vi "database_path.vi"(10 "部位":string, 11 "产品序号":string) -> (2 "database path":path)   [LabVIEW 2018]
panel:
  out "添加的路径":path
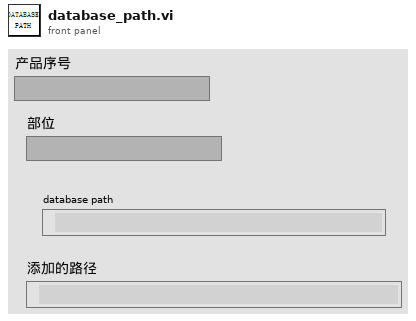
[diagram p1: front panel]
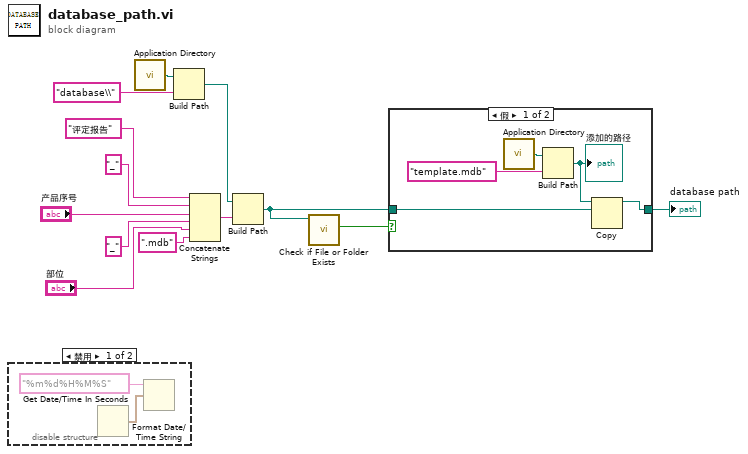
[diagram p0: block diagram]
diagram:
  n1 = disable-structure shown="禁用" {
    frame Disabled {
      n2 = Get Date/Time In Seconds() -> (seconds since 1Jan1904=w15:timestamp)
      n3 = Format Date/Time String(time format string (%c)="%m%d%H%M%S" ("时间格式字符串(%c)"), seconds (now)=w15) -> ()  [unwired: 1 in, 1 out]
    }
    frame Enabled {
    }
  }
  n4 = call <vilib>:"Application Directory.vi"() -> ("Application Directory"=w10:path)
  n5 = Build Path(base path=w10, name or relative path="database\\" ("名称或相对路径")) -> (appended path=w8:path)
  n6 = Concatenate Strings("评定报告" ("字符串"), "_" ("名称或相对路径"), "产品序号", "_" ("名称或相对路径"), "部位", ".mdb" ("字符串")) -> (w7:string)
  n7 = Build Path(base path=w8, name or relative path=w7) -> (appended path=w12:path)
  n8 = call <vilib>:"Check if File or Folder Exists.vi"("path"=w12) -> ("file or folder exists?"=w11:bool)  [unwired: 8 in, 2 out]
  n9 = case shown="假" w11 {
    tunnel: [w20 w21] -> w13
    tunnel: w12 -> [w19 w21]
    frame False {
      n10 = call <vilib>:"Application Directory.vi"() -> ("Application Directory"=w18:path)
      n11 = Build Path(base path=w18, name or relative path="template.mdb" ("名称或相对路径")) -> (appended path=w17:path)
      "添加的路径" <- w17
      n12 = Copy(10:w19, 11:w17) -> (3:w20:path)  [unwired: 3 in, 2 out]
    }
    frame True {
    }
  }
  "database path" <- w13
